vi "Update_Ch_Discription_server.vi"(1 "Mode":T7(ring), 2 "Client HD name":string="G3_3 HD", 3 "Channels to update In":T1[](array[typedef]) {"Duty" format="%.0b"; "D" format="%#_5g"; "C" format="%#_5g"; "B" format="%#_5g"; "A" format="%#_5g"}) -> (0 "Channels to update Out":T1[](array[typedef]) {"Duty" format="%.0b"; "D" format="%#_5g"; "C" format="%#_5g"; "B" format="%#_5g"; "A" format="%#_5g"})   [LabVIEW 2012]
uses:
  ADAM Client/Sub VIs/ADAM Controls/Ch_description_ADAM.ctl
  ADAM Client/Sub VIs/ADAM Controls/Module_type_ADAM.ctl
  ADAM Client/Sub VIs/ADAM Controls/Function_ADAM.ctl
  ADAM Client/Sub VIs/ADAM Controls/Channel_State.ctl
  ADAM Client/Sub VIs/ADAM Controls/Calib_type_ADAM.ctl
  ADAM Client/Sub VIs/ADAM Controls/Address.ctl
  ADAM_Global.vi
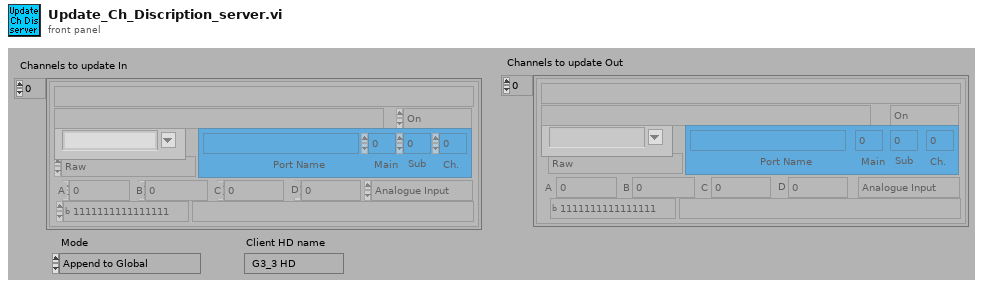
[diagram p1: front panel]
types:
  T1 = typedef "Ch_description_ADAM.ctl" = cluster{"Ch Name":string, "Type":T2, "Function":T3, "Ch State":T4, "Calibration type":T5, "A":dbl, "B":dbl, "C":dbl, "D":dbl, "Comments":string, "Address":T6, "String":string, "Duty":u16}
  T2 = typedef "Module_type_ADAM.ctl" = string
  T3 = typedef "Function_ADAM.ctl" = enum16{"Analogue Input", "Digital Input", "Event counter", "Event rate", "Analogue Output", "Digital Output", "Relay Output"}
  T4 = typedef "Channel_State.ctl" = enum16{"On", "Off", "Always On", "Always Off"}
  T5 = typedef "Calib_type_ADAM.ctl" = enum16{"Raw", "Bx + A", "Cx^2 + Bx + A", "Dx^3 + Cx^2 + Bx + A", "In Band", "Hi-Tec Q", "Hi-Tec M_dot", "Text"}
  T6 = typedef "Address.ctl" = cluster{"Main":i32, "Ch.":i32, "Sub":i32, "Port Name":string}
  T7 = enum16{"Append to Global", "Read Global then Clear"}
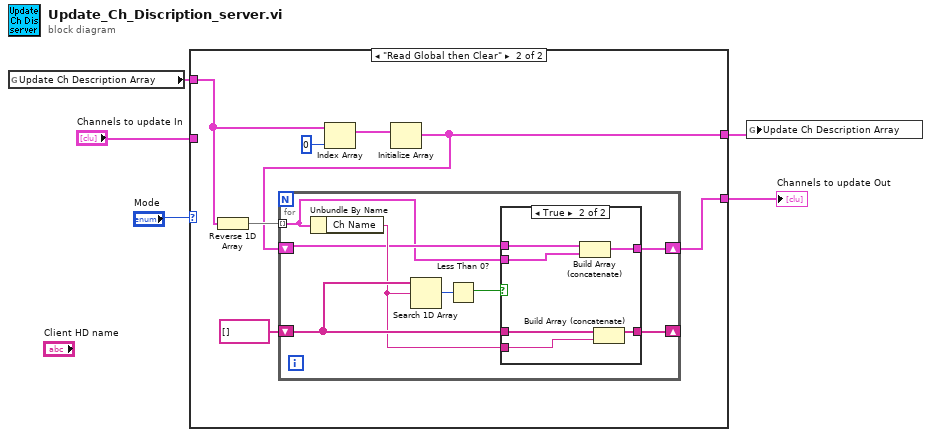
[diagram p0: block diagram]
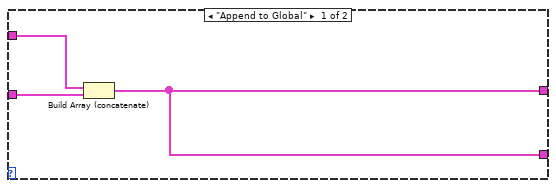
[diagram p2: hidden frame]
diagram:
  n1 = global read "ADAM_Global.vi" "Update Ch Description Array"() -> (w3:T1[])
  n2 = case shown="\"Read Global then Clear\"" "Mode" {
    tunnel: w3 -> [w8 w13]
    tunnel: "Channels to update In" -> [w7 _]
    tunnel: [w6 w11] -> w5
    tunnel: [w6 w10] -> w1
    frame "Append to Global" {
      n3 = Build Array (concatenate)(w8, w7) -> (w6:T1[])
    }
    frame "Read Global then Clear" {
      n4 = Reverse 1D Array(array=w13) -> (reversed array=w12:T1[])
      n5 = Index Array(array=w13, index=0) -> (element=w14:T1)
      n6 = Initialize Array(w14) -> (w11:T1[])  [unwired: 1 out]
      n7 = for {
        tunnel: w12 -> [w16] mode=indexing
        shift-right: [w20] -> _
        shift-left: string[] [] -> [w21]
        shift-right: [w17] -> w10
        shift-left: w11 -> [w18]
        n8 = Unbundle By Name(w16) -> ("Ch Name"=w19:string)
        n9 = Search 1D Array(1D array=w21, element=w19) -> (index of element=w23:i32)  [unwired: 1 out]
        n10 = Less Than 0?(x=w23) -> (x < 0?=w22:bool)
        n11 = case shown="True" w22 {
          tunnel: w21 -> [w24 w31]
          tunnel: [w24 w30] -> w20
          tunnel: w19 -> [_ w29]
          tunnel: w18 -> [w25 w28]
          tunnel: [w25 w27] -> w17
          tunnel: w16 -> [_ w26]
          frame False {
          }
          frame True {
            n12 = Build Array (concatenate)(w28, w26) -> (w27:T1[])
            n13 = Build Array (concatenate)(w31, w29) -> (w30:string[])
          }
        }
      }
    }
  }
  "Channels to update Out" <- w1
  n14 = global write "ADAM_Global.vi" "Update Ch Description Array"(w5) -> ()
